vi "Step done.vi"(8 "Auto cycle checks in":T2, 11 "Auto cycle step":T1) -> (0 "Auto cycle checks out":T2)   [LabVIEW 2017, in "Auto cycle.lvlib"]
uses:
  Auto cycle.lvlib
  Checks.ctl
  Steps.ctl
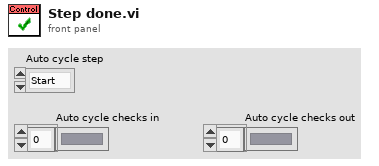
[diagram p1: front panel]
types:
  T1 = typedef "Auto cycle.lvlib/Steps.ctl" = enum16{"Start", "Setup spectrum", "Setup monochromator", "Setup colour wheel", "Move shutter", "Collect data", "Process A or B test", "A-B processing, stitching", "Return shutter"}
  T2 = typedef "Auto cycle.lvlib/Checks.ctl" = bool[]
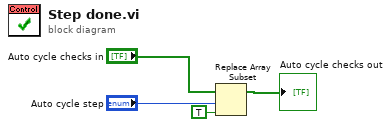
[diagram p0: block diagram]
diagram:
  n1 = Replace Array Subset(array="Auto cycle checks in", new element=TRUE ("new element/subarray"), index="Auto cycle step") -> (→"Auto cycle checks out":T2)
